vi "Get Velocity from Wheels.vi"   [LabVIEW 2017, in "NI_Robotics_Steering Frame.lvclass"]
doc: "Calculates the steering frame velocity or arc velocity required to best satisfy the state of each wheel. You can read data for each wheel from wheel motors or specify the wheel data manually. You must manually select the polymorphic instance to use."
uses:
  <vilib>/robotics/Steering/Steering Frame/NI_Robotics_Steering Frame.lvclass
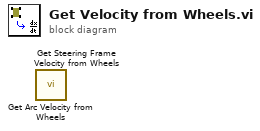
[diagram p0: block diagram]
diagram:
  n1 = call <vilib>:"Get Arc Velocity from Wheels.vi"() -> ()  [unwired: 8 in, 4 out]
  n2 = call <vilib>:"Get Steering Frame Velocity from Wheels.vi"() -> ()  [unwired: 8 in, 4 out]
